vi "addToUndo.vi"(8 "error in (no error)":errorcluster, 11 "ScriptEditorV2 in":refnum<class "ScriptEditorV2.lvclass">) -> (0 "error out":errorcluster, 3 "ScriptEditorV2 out":refnum<class "ScriptEditorV2.lvclass">)   [LabVIEW 2011, in "Views.lvlib" / "ScriptEditor.lvlib" / "ScriptEditorV2.lvclass"]
uses:
  ScriptEditorV2.lvclass
  ScriptEditorV2.lvclass/ScriptEditorV2.ctl
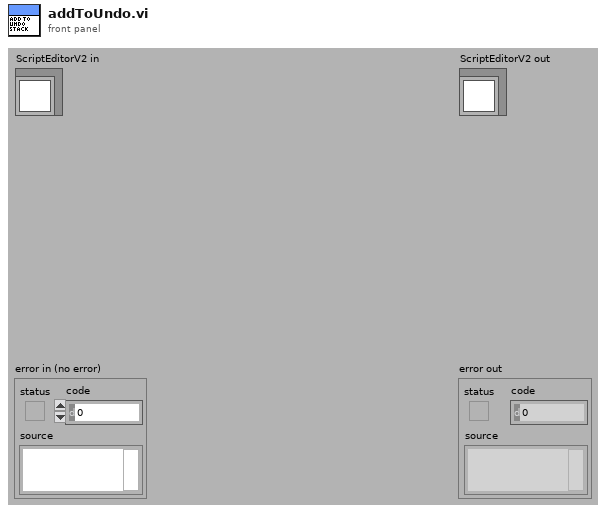
[diagram p1: front panel]
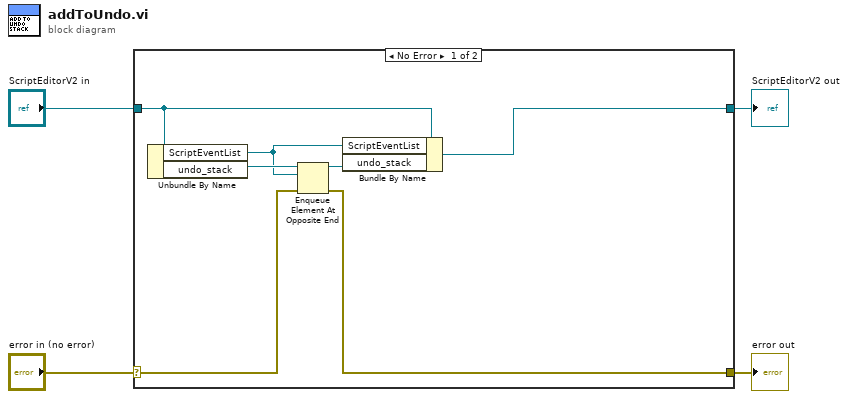
[diagram p0: block diagram]
diagram:
  n1 = case shown="No Error" "error in (no error)" {
    selector: "error in (no error)" -> [w10 w13]
    tunnel: [w9 w13] -> w3
    tunnel: [w5 w12] -> w1
    tunnel: "ScriptEditorV2 in" -> [w6 w12]
    frame No Error {
      n2 = Unbundle By Name(w6) -> ("ScriptEventList"=w7:refnum<class "ScriptEventList.lvclass">, "undo_stack"=w11:refnum<queue>)
      n3 = Enqueue Element At Opposite End(queue=w11, element=w7, error in (no error)=w10) -> (queue out=w8:refnum<queue>, error out=w9:errorcluster)  [unwired: 1 in, 1 out]
      n4 = Bundle By Name(cluster=w6, "ScriptEventList"=w7, "undo_stack"=w8) -> (w5:refnum<class "ScriptEditorV2.lvclass">)
    }
    frame Error {
    }
  }
  "error out" <- w3
  "ScriptEditorV2 out" <- w1
